vi "set_transformation_factors.vi"(8 "error in (no error)":errorcluster, 10 "transformation factors":dbl[unit][](array[numeric]), 11 "TrajectoryMG100122AODFrameScan in":refnum<class "TrajectoryMG100122AODFrameScan.lvclass">) -> (0 "error out":errorcluster, 3 "TrajectoryMG100122AODFrameScan out":refnum<class "TrajectoryMG100122AODFrameScan.lvclass">)   [LabVIEW 2010, in "TrajectoryMG100122AODFrameScan.lvclass"]
uses:
  TrajectoryMG100122AODFrameScan.lvclass
  TrajectoryMG100122AODFrameScan.lvclass/TrajectoryMG100122AODFrameScan.ctl
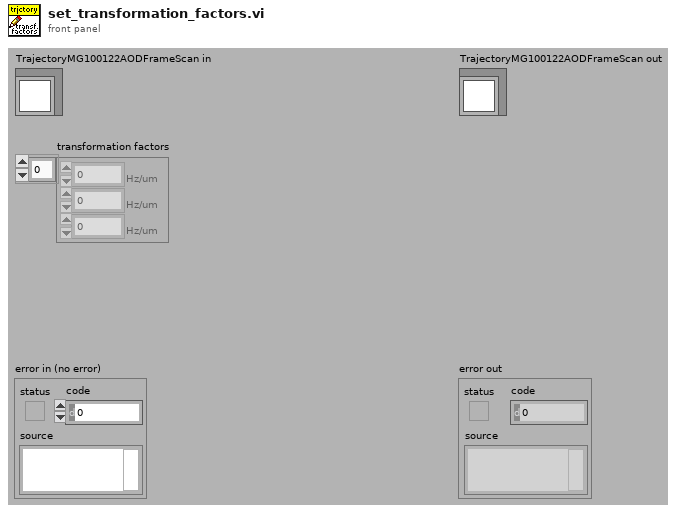
[diagram p1: front panel]
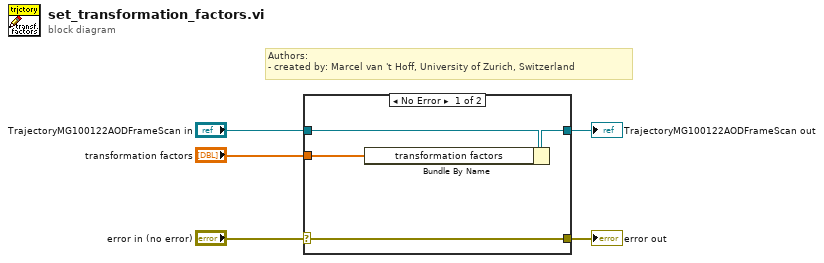
[diagram p0: block diagram]
diagram:
  # "Authors: \n- created by: Marcel van 't Hoff, University of Zurich, Switzerland"
  n1 = case shown="No Error" "error in (no error)" {
    selector: "error in (no error)" -> [w9 w10]
    tunnel: [w9 w10] -> w4
    tunnel: [w7 w11] -> w2
    tunnel: "TrajectoryMG100122AODFrameScan in" -> [w8 w11]
    tunnel: "transformation factors" -> [w6 _]
    frame No Error {
      n2 = Bundle By Name(cluster=w8, "transformation factors"=w6) -> (w7:refnum<class "TrajectoryMG100122AODFrameScan.lvclass">)
    }
    frame Error {
    }
  }
  "error out" <- w4
  "TrajectoryMG100122AODFrameScan out" <- w2
